vi "Open Log Dir.vi"(8 "error in (no error)":errorcluster) -> (0 "error out":errorcluster)   [LabVIEW 2014]
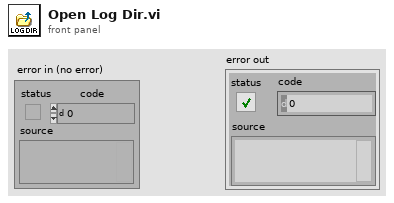
[diagram p1: front panel]
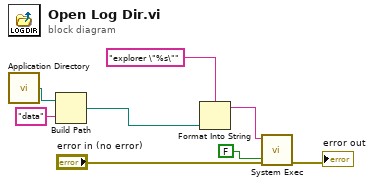
[diagram p0: block diagram]
diagram:
  n1 = call <vilib>:"Application Directory.vi"() -> ("Application Directory"=w3:path)
  n2 = Build Path(base path=w3, name or relative path="data") -> (appended path=w1:path)
  n3 = Format Into String(format string="explorer \"%s\"", w1) -> (resulting string=w4:string)  [unwired: 2 in, 1 out]
  n4 = call <vilib>:"System Exec.vi"("run minimized? (F)"=FALSE, "error in (no error)"="error in (no error)", "command line"=w4) -> ("error out"=→"error out":errorcluster)  [unwired: 5 in, 3 out]
